vi "Dock.vi"(0 "LV MDI.lvclass":refnum<class "LV MDI.lvclass">, 5 "Undock?":bool, 11 "error in (no error)":errorcluster) -> (4 "LV MDI.lvclass":refnum<class "LV MDI.lvclass">, 15 "error out":errorcluster)   [LabVIEW 2016, in "LV MDI.lvclass"]
doc: "Dock and Undock child window from MDI panel."
uses:
  LV MDI.lvclass
  LV MDI.lvclass/LV MDI.ctl
  user32.dll
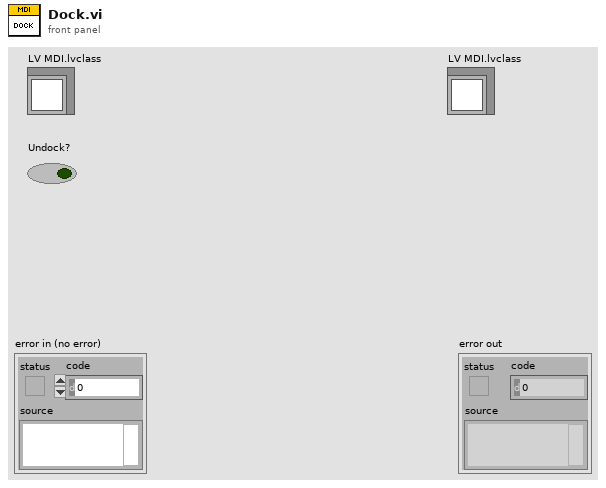
[diagram p1: front panel]
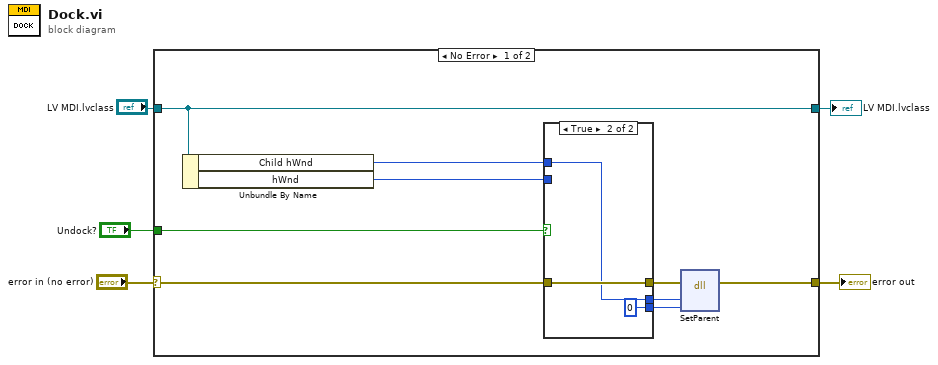
[diagram p0: block diagram]
diagram:
  n1 = case shown="No Error" "error in (no error)" {
    selector: "error in (no error)" -> [w14 w22]
    tunnel: [w10 w22] -> w4
    tunnel: [w7 w21] -> w2
    tunnel: "LV MDI.lvclass" -> [w7 w21]
    tunnel: "Undock?" -> [w12 _]
    frame No Error {
      n2 = Unbundle By Name(w7) -> ("Child hWnd"=w6:u32, "hWnd"=w11:i32)
      n3 = case shown="True" w12 {
        tunnel: w14 -> [w17 w20]
        tunnel: [w17 w20] -> w13
        tunnel: [w16 w19] -> w9
        tunnel: [w15 0 ("hWnd")] -> w8
        tunnel: w6 -> [w16 w19]
        tunnel: w11 -> [w15 _]
        frame False {
        }
        frame True {
        }
      }
      n4 = dll-call lib="user32.dll" fn="SetParent"(error in=w13, "Child"=w9, "NewParent"=w8) -> (error out=w10:errorcluster)  [unwired: 5 in, 1 out]
    }
    frame Error {
    }
  }
  "error out" <- w4
  "LV MDI.lvclass" <- w2
